vi "open.vi"(0 "object in":refnum<class "tcp_work.lvclass">, 1 "input":T1={"IP"="", "PORT"="", "VISA resource name"="", "baud rate (9600)"=115200, "data bits (8)"=8, "parity (0:none)"=enum."None", "timeout (10sec)"=10000} {"data bits (8)" min=5 max=8 step=1}, 5 "error in (no error)":errorcluster) -> (14 "object out":refnum<class "tcp_work.lvclass">, 19 "error out":errorcluster)   [LabVIEW 2016, in "tcp_work.lvclass"]
uses:
  tcp_work.lvclass
  tcp_work.lvclass/tcp_work.ctl
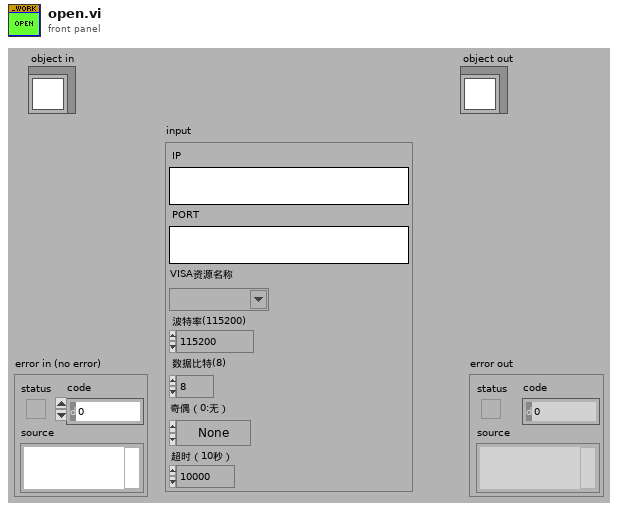
[diagram p1: front panel]
types:
  T1 = cluster{"IP":string, "PORT":string, "VISA resource name":refnum<visa-resource-name>, "baud rate (9600)":u32, "data bits (8)":u16, "parity (0:none)":enum16{"None", "Odd", "Even", "Mark", "Space"}, "timeout (10sec)":u32}
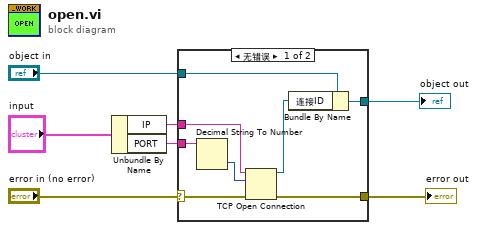
[diagram p0: block diagram]
diagram:
  n1 = Unbundle By Name("input") -> ("IP"=w2:string, "PORT"=w1:string)
  n2 = case shown="无错误" "error in (no error)" {
    selector: "error in (no error)" -> [w9 w17]
    tunnel: [w8 w17] -> w6
    tunnel: [w14 w16] -> w4
    tunnel: "object in" -> [w15 w16]
    tunnel: w2 -> [w12 _]
    tunnel: w1 -> [w11 _]
    frame No Error {
      n3 = Decimal String To Number(string=w11) -> (number=w13:i32)  [unwired: 2 in, 1 out]
      n4 = TCP Open Connection(address=w12, remote port or service name=w13, error in (no error)=w9) -> (connection ID=w10:refnum<k5>, error out=w8:errorcluster)  [unwired: 2 in]
      n5 = Bundle By Name(cluster=w15, "连接ID"=w10) -> (w14:refnum<class "tcp_work.lvclass">)
    }
    frame Error {
    }
  }
  "error out" <- w6
  "object out" <- w4
